vi "Program_2.vi"() -> ()   [LabVIEW 2024]
uses:
  Program_1_Global.vi
panel:
  out "(m, n)":dbl(graph)
  out "Min":dbl(graph)
  out "Max":dbl(graph)
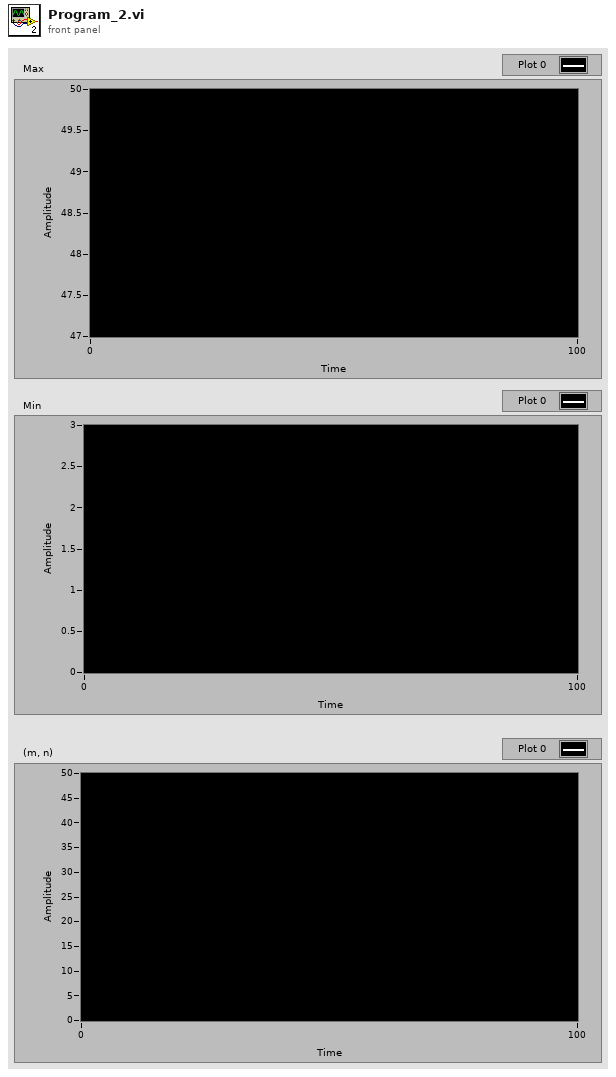
[diagram p1: front panel]
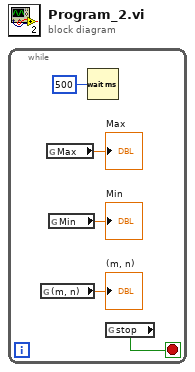
[diagram p0: block diagram]
diagram:
  n1 = while {
    stop <- w5 stop-if-true
    n2 = global read "Program_1_Global.vi" "(m, n)"() -> (→"(m, n)":dbl)
    n3 = global read "Program_1_Global.vi" "Max"() -> (→"Max":dbl)
    n4 = global read "Program_1_Global.vi" "Min"() -> (→"Min":dbl)
    n5 = Wait (ms)(milliseconds to wait=u32 500) -> ()  [unwired: 1 out]
    n6 = global read "Program_1_Global.vi" "stop"() -> (w5:bool)
  }
